vi "subvi_ByteArrayToPointer.vi"(8 "error in (no error)":errorcluster, 11 "Byte Array In":u8[](array[numeric])) -> (0 "error out":errorcluster, 2 "Size":i32, 3 "Pointer":i32)   [LabVIEW 2013]
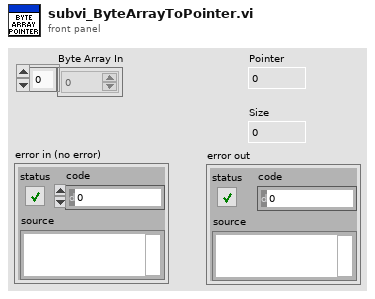
[diagram p1: front panel]
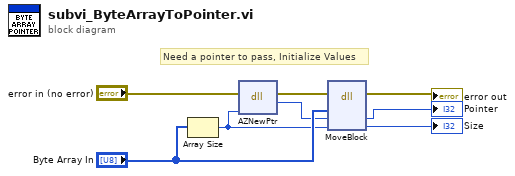
[diagram p0: block diagram]
diagram:
  # "Need a pointer to pass, Initialize Values"
  n1 = Array Size(array="Byte Array In") -> (size(s)=w5:i32)
  n2 = dll-call lib="LabVIEW" fn="AZNewPtr"(error in="error in (no error)", "size"=w5) -> (error out=w6:errorcluster, "ptr"=w3:i32)  [unwired: 3 in, 1 out]
  n3 = dll-call lib="LabVIEW" fn="MoveBlock"(error in=w6, "src"="Byte Array In", "dest"=w3, "size"=w5) -> (error out=→"error out":errorcluster, "dest"=→"Pointer":i32, "size"=→"Size":i32)  [unwired: 4 in, 1 out]
